vi "TwoSignalEdgeSeparation example.vi"() -> ()   [LabVIEW 2014]
uses:
  <vilib>/DAQmx/create/channels.llb/DAQmx Create Channel (CO-Pulse Generation-Frequency).vi
  <vilib>/DAQmx/configure/trigger.llb/DAQmx Start Trigger (Digital Edge).vi
  <vilib>/DAQmx/create/channels.llb/DAQmx Create Channel (CI-Count Edges).vi
  <vilib>/DAQmx/read.llb/DAQmx Read (Counter DBL 1Chan 1Samp).vi
  <vilib>/DAQmx/configure/timing.llb/DAQmx Timing (Implicit).vi
  <resource>/objmgr/daqmx.rc
  <vilib>/DAQmx/create/channels.llb/DAQmx Create Channel (CI-Two Edge Separation).vi
panel:
  in  "frequency":dbl=80000000.0
  in  "stop":bool
  out "time difference (s)":dbl
  in  "2nd Signal Active State":i32(ring)=10192 items=["High"=10192, "Low"=10214]
  in  "1st Signal Edge":i32(ring)=10280 items=["Rising"=10280, "Falling"=10171]
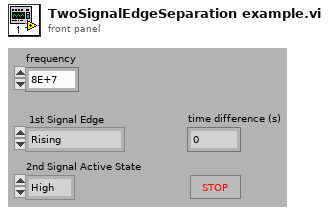
[diagram p1: front panel]
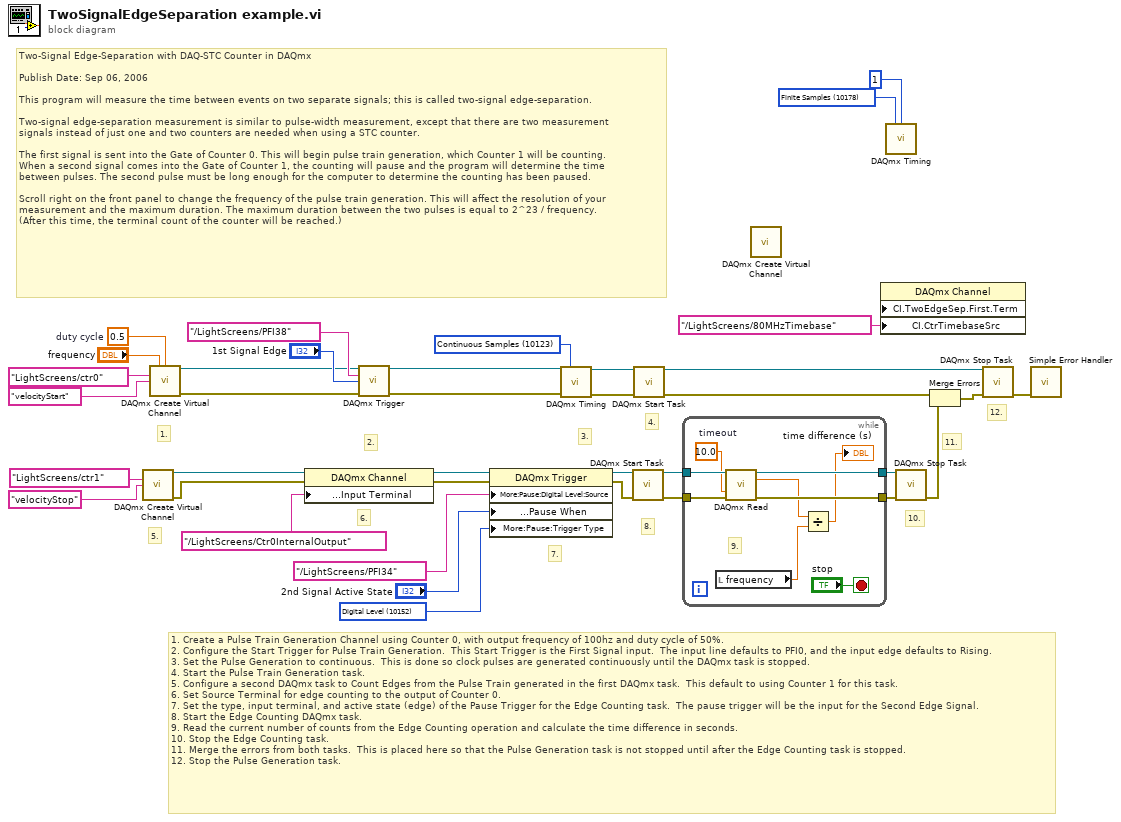
[diagram p0: block diagram]
diagram:
  w2 = 10178 items=["Finite Samples"=10178, "Continuous Samples"=10123, "Hardware Timed Single Point"=12522] ("sample mode")
  w17 = 10123 items=["Finite Samples"=10178, "Continuous Samples"=10123] ("sample mode")
  w19 = 10152 items=["Analog Level"=10101, "Analog Window"=10103, "Digital Level"=10152, "None"=10230] ("Pause.TrigType")
  w37 = 0.5  # duty cycle
  # "Two-Signal Edge-Separation with DAQ-STC Counter in DAQmx\n\nPublish Date: Sep 06, 2006\n\nThis program will measure the time between events on two separate signals; this is called two-signal edge-separation.\n\nTwo-signal edge-separation measurement is similar to pulse-width measurement, except that there are two measurement \nsignals instead of just one and two counters are needed when using a STC counter.\n\nThe first signal is sent into the Gate of Counter 0. This will begin pulse train generation, which Counter 1 will be counting. \nWhen a second signal comes into the Gate of Counter 1, the counting will pause and the program will determine the time \nbetween pulses. The second pulse must be long enough for the computer to determine the counting has been paused.\n\nScroll right on the front panel to change the frequency of the pulse train generation. This will affect the resolution of your \nmeasurement and the maximum duration. The maximum duration between the two pulses is equal to 2^23 / frequency. \n(After this time, the terminal count of the counter will be reached.)"
  # "12."
  # "11."
  # "10."
  # "8."
  # "7."
  # "6."
  # "5."
  # "4."
  # "3."
  # "2."
  # "1."
  # "1. Create a Pulse Train Generation Channel using Counter 0, with output frequency of 100hz and duty cycle of 50%.\n2. Configure the Start Trigger for Pulse Train Generation.  This Start Trigger is the First Signal input.  The input line defaults to PFI0, and the input edge defaults to Rising.\n3. Set the Pulse Generation to continuous.  This is done so clock pulses are generated continuously until the DAQmx task is stopped.\n4. Start the Pulse Train Generation task.\n5. Configure a second DAQmx task to Count Edges from the Pulse Train generated in the first DAQmx task.  This default to using Counter 1 for this task.\n6. Set Source Terminal for edge counting to the output of Counter 0.\n7. Set the type, input terminal, and active state (edge) of the Pause Trigger for the Edge Counting task.  The pause trigger will be the input for the Second Edge Signal.\n8. Start the Edge Counting DAQmx task.\n9. Read the current number of counts from the Edge Counting operation and calculate the time difference in seconds.\n10. Stop the Edge Counting task.\n11. Merge the errors from both tasks.  This is placed here so that the Pulse Generation task is not stopped until after the Edge Counting task is stopped.\n12. Stop the Pulse Generation task."
  n1 = call-poly <vilib>:"DAQmx Create Virtual Channel.vi"("counter"=tag "LightScreens/ctr1" ("counter2"), "name to assign"="velocityStop") -> ("task out"=w13:refnum<k21>, "error out"=w11:errorcluster)  [unwired: 12 in]
  n2 = call-poly <vilib>:"DAQmx Create Virtual Channel.vi"("frequency"="frequency", "duty cycle"=w37, "counter"=tag "LightScreens/ctr0" ("counter1"), "name to assign"="velocityStart") -> ("task out"=w9:refnum<k21>, "error out"=w8:errorcluster)  [unwired: 10 in]
  n3 = property class="DAQmx Channel"(reference=w13, error in=w11, "Counter Input:Count Edges:Input Terminal"=tag "/LightScreens/Ctr0InternalOutput" ("CI.CountEdges.Term")) -> (reference out=w12:refnum<k21>, error out=w10:errorcluster)
  n4 = call-poly <vilib>:"DAQmx Trigger.vi"("task/channels in"=w9, "source"=tag "/LightScreens/PFI38", "edge"="1st Signal Edge", "error in"=w8) -> ("task out"=w18:refnum<k21>, "error out"=w16:errorcluster)  [unwired: 10 in]
  n5 = property class="DAQmx Trigger"(reference=w12, error in=w10, "More:Pause:Digital Level:Source"=tag "/LightScreens/PFI34" ("Pause.DigLvl.Src"), "More:Pause:Digital Level:Pause When"="2nd Signal Active State", "More:Pause:Trigger Type"=w19) -> (reference out=w30:refnum<k21>, error out=w29:errorcluster)
  n6 = call-poly <vilib>:"DAQmx Timing.vi"("task/channels in"=w18, "sample mode"=w17, "error in"=w16) -> ("task out"=w14:refnum<k21>, "error out"=w15:errorcluster)  [unwired: 11 in]
  n7 = call <vilib>:"DAQmx Start Task.vi"("task/channels in"=w30, "error in"=w29) -> ("task out"=w22:refnum<k21>, "error out"=w21:errorcluster)  [unwired: 12 in]
  n8 = call <vilib>:"DAQmx Start Task.vi"("task/channels in"=w14, "error in"=w15) -> ("task out"=w7:refnum<k21>, "error out"=w27:errorcluster)  [unwired: 12 in]
  n9 = while {
    tunnel: [w46] -> w24
    tunnel: [w45] -> w23
    tunnel: w22 -> [w44]
    tunnel: w21 -> [w40]
    stop <- "stop" stop-if-true
    w38 = 10.0  # timeout
    # "9."
    n10 = local read "frequency"() -> (w39:dbl)
    n11 = call-poly <vilib>:"DAQmx Read.vi"("task/channels in"=w44, "timeout"=w38, "error in"=w40) -> ("task out"=w46:refnum<k21>, "data"=w41:dbl, "error out"=w45:errorcluster)  [unwired: 10 in]
    n12 = Divide(x=w41, y=w39) -> (x/y=→"time difference (s)":dbl)
  }
  n13 = call-poly <vilib>:"DAQmx Create Virtual Channel.vi"() -> ()  [unwired: 14 in, 2 out]
  n14 = property class="DAQmx Channel" props=["CI.TwoEdgeSep.First.Term", "CI.CtrTimebaseSrc"]("CI.CtrTimebaseSrc"=tag "/LightScreens/80MHzTimebase") -> ()  [unwired: 3 in, 2 out]
  n15 = call-poly <vilib>:"DAQmx Timing.vi"("sample mode"=w2, "samples per channel"=1) -> ()  [unwired: 12 in, 2 out]
  n16 = call <vilib>:"DAQmx Stop Task.vi"("task/channels in"=w24, "error in"=w23) -> ("error out"=w26:errorcluster)  [unwired: 12 in, 1 out]
  n17 = Merge Errors(w27, w26) -> (w25:errorcluster)
  n18 = call <vilib>:"DAQmx Stop Task.vi"("task/channels in"=w7, "error in"=w25) -> ("error out"=w28:errorcluster)  [unwired: 12 in, 1 out]
  n19 = call <vilib>:"Simple Error Handler.vi"("error in (no error)"=w28) -> ()  [unwired: 4 in, 5 out]
